vi "Convert to Snake Case.vi"(8 "error in (no error)":errorcluster, 10 "All Upper Case? (F)":bool, 11 "Input String":string) -> (0 "error out":errorcluster, 3 "Output String":string)   [LabVIEW 2015, in "Case Manipulation.lvlib"]
doc: "Introduction:\nWe often remove the spaces between words because programs of different sorts reserve the space (‘ ’) character for special purposes. Because the space character is reserved, we cannot use it to represent a concept that we express in our human language with multiple words.\nSnake Case:\nThis style, when capitalized, is often used as a convention in declaring constants in many languages. When lower cased, it is used conventionally in declaring database field names."
uses:
  Case Manipulation.lvlib
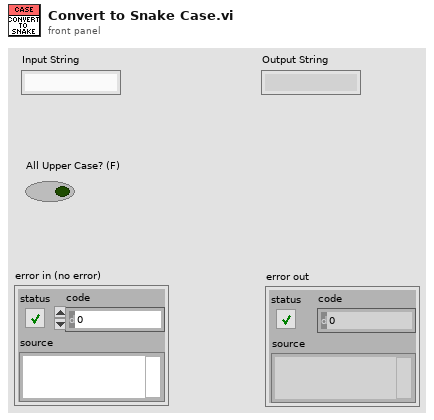
[diagram p1: front panel]
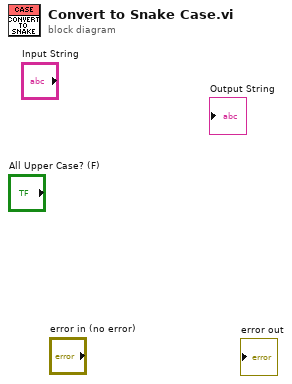
[diagram p0: block diagram]
diagram:
